vi "InitDevice.vi"(8 "error in (no error)":errorcluster, 11 "Acq Thread Data in":T1) -> (0 "error out":errorcluster, 3 "Acq Thread Data out":T1)   [LabVIEW 2019]
uses:
  Typedefs/Acquisition Thread/#cluster_AcqThreadData.ctl
  <vilib>/MagicBox/Device/Arduino/Arduino.lvclass
  <vilib>/MagicBox/Peripherals/POX/POX.lvclass
  Typedefs/Acquisition Thread/#enum_AcqThreadState.ctl
  Typedefs/#cluster_GUIRefs.ctl
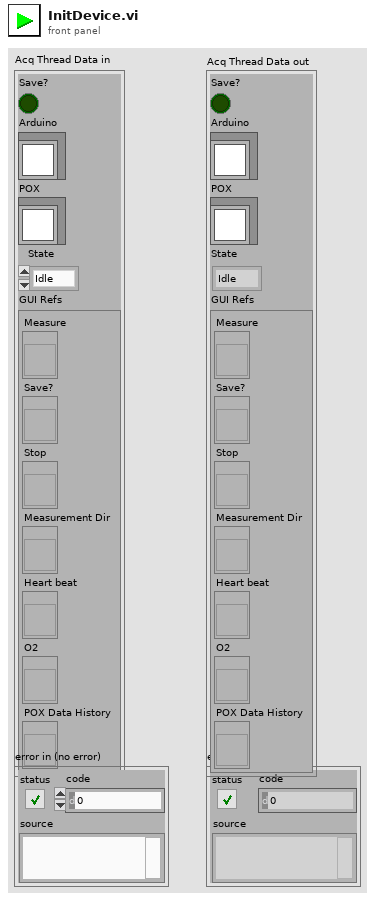
[diagram p1: front panel]
types:
  T1 = typedef "#cluster_AcqThreadData.ctl" = cluster{"Save?":bool, "Arduino":refnum<class "Arduino.lvclass">, "POX":refnum<class "POX.lvclass">, "State":T2, "GUI Refs":T3}
  T2 = typedef "#enum_AcqThreadState.ctl" = enum16{"Idle", "Operate", "Error"}
  T3 = typedef "#cluster_GUIRefs.ctl" = cluster{"Measure":refnum<vi>, "Save?":refnum<vi>, "Stop":refnum<vi>, "Measurement Dir":refnum<vi>, "Heart beat":refnum<vi>, "O2":refnum<vi>, "POX Data History":refnum<vi>}
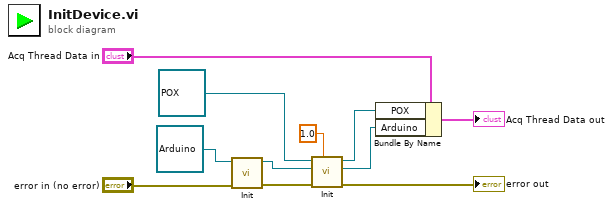
[diagram p0: block diagram]
diagram:
  n1 = call-dynamic "Init.vi"("error in (no error)"="error in (no error)", "Arduino in"=refnum<class "Arduino.lvclass"> refnum) -> ("error out"=w7:errorcluster, "Arduino out"=w6:refnum<class "Arduino.lvclass">)  [unwired: 8 in]
  n2 = call-dynamic "Init.vi"("Sample Rate (n/s)"=1.0, "error in (no error)"=w7, "Arduino in"=w6, "POX in"=refnum<class "POX.lvclass"> refnum) -> ("error out"=→"error out":errorcluster, "Arduino out"=w3:refnum<class "Arduino.lvclass">, "POX out"=w4:refnum<class "POX.lvclass">)  [unwired: 5 in]
  n3 = Bundle By Name(cluster="Acq Thread Data in", "POX"=w4, "Arduino"=w3) -> (→"Acq Thread Data out":T1)
